vi "BeadTrackerMain.vi"() -> ()   [LabVIEW 2011]
uses:
  qtrk/QTrkLVBinding/QTrkLocalizationType.ctl
  Main/Typedefs/MeasureConfigType.ctl
  Main/Typedefs/MeasureConfigOutputMode.ctl
  qtrk/QTrkLVBinding/QTrkSettings.ctl
  Main/Typedefs/TrackingConfigType.ctl
  qtrk/QTrkLVBinding/QTrkZCommandType.ctl
  Main/ExperimentProgram/ExperimentProgramType.ctl
  Main/ExperimentProgram/ExProgCommandType.ctl
  Main/ExperimentProgram/ExProgCommandEnumType.ctl
  Main/Motors/MotorAxisEnum.ctl
  Main/Motors/MotorPosType.ctl
  Main/Typedefs/XYf.ctl
  Main/Motors/MotorPosFlagsType.ctl
  Main/Camera/GenericCameraConfigType.ctl
  <vilib>/vision/Image Controls.llb/IMAQ Image.ctl
  qtrk/QTrkLVBinding/ResultManagerInstance.ctl
  Main/Typedefs/CmdEnum_UserInterfaceCmd.ctl
  Main/Typedefs/CmdEnum_CameraFrameType.ctl
  Main/GlobalVariables.vi
  Main/Tracking/SemaphoreResultManager.vi
  <vilib>/vision/NI_Vision_Development_Module.lvlib
  <vilib>/Analysis/NI_AALBase.lvlib
panel:
  out "Buffer Image":T1
  in  "Default measure config":T2={"Bead locations"=[{"X"=0, "Y"=0}], "ROI"=80, "Experiment base path"=path "", "Image output subdir"="images", "Output mode"=enum."Track", "Traces output subdir"="traces", "QTrk Settings"={"Image width"=150, "Image height"=150, "Number of threads (CPU based)"=-1, "CUDA Device"=-2, "COM Background correction factor"=0.0, "ZLUT MinRadius"=2.0, "ZLUT Radial sample density"=2.0, "ZLUT Angular sample density"=0.7, "ZLUT ROI Coverage"=1.0, "QI Iterations"=3, "QI MinRadius"=2.0, "QI Radial sample density"=2.0, "QI Angular sample density"=0.7, "QI ROI Coverage"=1.0, "QI Angular Step \nIteration Factor"=1.2, "XCOR Profile Length"=1, "XCOR Profile Width"=128, "XCOR Iterations"=32, "Gaussian 2D Fit Iterations"=2, "Gaussian 2D Sigma (pixels)"=3.0, "Downsample"=0}, "Tracking Config"={"Number of steps"=100, "ZLUT stepsize (um)"=0.05, "Z correction factor"=0.88, "Start piezo Z (um)"=0.0, "Pixel size (nm)"=146.0, "2D Localization Type"=enum."Quadrant Interpolation", "Z Command (None)"=enum."ComputeZ", "Z Piezo scale"=FALSE, "ZLUT Building\nimages per frame"=0}, "Experiment Name"="test", "Program"={"Commands"=[], "Motor Axis accuracy conditions"={"Magnet Z"=0.0, "Magnet rotation"=0.0, "Camera"={"X"=0.0, "Y"=0.0}, "Piezo XY"={"X"=0.0, "Y"=0.0}, "Piezo Z"=0.0, "Coil XY"={"X"=0.0, "Y"=0.0}}, "Axis flags"={"Magnet Z"=FALSE, "Magnet rotation"=FALSE, "Camera"={"X"=FALSE, "Y"=FALSE}, "Piezo XY"={"X"=FALSE, "Y"=FALSE}, "Piezo Z"=FALSE, "Coil XY"={"X"=FALSE, "Y"=FALSE}}}, "ZLUT"=[], "Camera settings"={"Framerate (Hz)"=60, "Exposure time (us)"=5000, "Image size"={"Width"=1280, "Height"=1024}, "Number of buffers"=30}, "Experiment Script"="", "Max frames in memory"=100000, "Save traces as binary"=FALSE, "Pixel Calibration Gain Image"="camera_calib_gain.bin", "Pixel Calibration Offset Image"="camera_calib_offset.bin", "Use pixel calibration images"=FALSE, "Internal camera settings"="", "Trace write interval"=100} {"QTrk Settings"."QI ROI Coverage" format="%_2g"; "QTrk Settings"."QI MinRadius" format="%.2f"; "QTrk Settings"."QI Angular sample density" format="%.3f"; "QTrk Settings"."QI Radial sample density" format="%.2f"; "QTrk Settings"."ZLUT Radial sample density" format="%.2f"; "QTrk Settings"."ZLUT MinRadius" format="%.2f"}
  out "Bead positions":cluster{"X":dbl, "Y":dbl}[](array[cluster])
  in  "Compute fisher accuracy":bool
  out "Offset":sgl[][](array[numeric])
  out "Normalized 1/Gain":sgl[][](array[numeric])
  out "Number of listeners":i32
  out "Running\nexperiment":bool
  out "Cam loop\nupdate speed":dbl
  in  "UpdateTraces":cluster{"ID":dbl}
  in  "UpdateLUT":cluster{"ID":dbl}
  in  "ImageOrResultViewTab":enum32{"Image", "Traces & LUT", "Message Log"}(tab)
  out "Image mean value":sgl(graph)
  in  "Hardware ROI index":i32
  out "Histogram":u32[](graph)
  out "Image":T1(plugin-control)
  out "Frame#":i32
  out "Framerate":dbl format="%#_1f"
  in  "Show image?":bool=TRUE
  in  "Histogram":bool
  out "Minimal Value":sgl
  out "Maximal Value":sgl
  in  "Save image":bool
  out "LUT minimum\nplane index":i32
  in  "Save LUT image":bool
  out "Bead image":u8[][](graph)
  in  "Start frame for trace display":i32(slide) max=9720 scale=0.0..3265.0
  in  "Reference bead#":i32 max=33
  in  "Subtract reference":bool
  in  "Discard bead":bool
  out "Bead XY":sgl[][](graph)
  in  "Bead index":i32 min=0 max=5
  out "Bead Z":sgl[](graph)
  out "Z Lookup Table":sgl[][](graph)
  in  "Number of frames to display":i32=1000 max=33
  out "Bead validity":dbl
  in  "Auto discard":bool
  in  "Minimum bead validity":dbl=1.0
  out "LUT minimum\nplane difference":dbl
  in  "LUT Inspect":bool
  out "Message Log":i32(listbox)
  out "ZLUT":sgl[][][](array[numeric])
  in  "UpdateUI":cluster{"ID":dbl}
  in  "Tab Control":T16(tab)
  out "Camera settings":variant
  in  "Camera settings":bool
  out "Expected location of beadlist:":path
  in  "Load beadlist":bool
  in  "Save beadlist":bool
  in  "ROI":i32=80
  in  "Select beads":bool
  out "Number of beads":i32
  out "LUT location":path
  in  "Load ZLUT":bool
  in  "Save ZLUT":bool
  in  "Save default settings":bool
  in  "Reload default settings":bool
  in  "2D Localization Type":T6
  in  "Pixel size (nm)":sgl=0.88
  in  "Set current piezo Z as start Z":bool
  in  "Edit QTrk settings":bool
  in  "ZLUT Start piezo Z":sgl=0.88
  in  "Number of steps":i32
  in  "Step size (um)":sgl
  in  "Z correction factor":sgl=0.88
  in  "Build ZLUT":bool
  in  "Select QTrk DLL":bool
  out "Settings location:":path
  in  "Use LUT scale for Z":bool=TRUE
  in  "Pixel calibration gain:":path
  in  "Pixel calibration offset:":path
  in  "Use gain/offset \ncorrection?":bool
  out "Mean":dbl format="%0.2f"
  out "Mean":dbl format="%0.2f"
  out "Max":sgl
  out "Min":sgl
  out "Max":sgl
  out "Min":sgl
  out "Gain image size":i32[](array[numeric])
  out "Offset image size":i32[](array[numeric])
  out "St Dev.":dbl format="%0.2f"
  out "St. Dev":dbl format="%0.2f"
  in  "stop":bool
  # "(used for commands with string parameters)"
  # "-2: Use all devices\n-1: Use best device"
  # "If the camera is giving multiple ROIs, this allows you to select the one that is displayed"
  # "Discard bead also discards bead results and bead ZLUT"
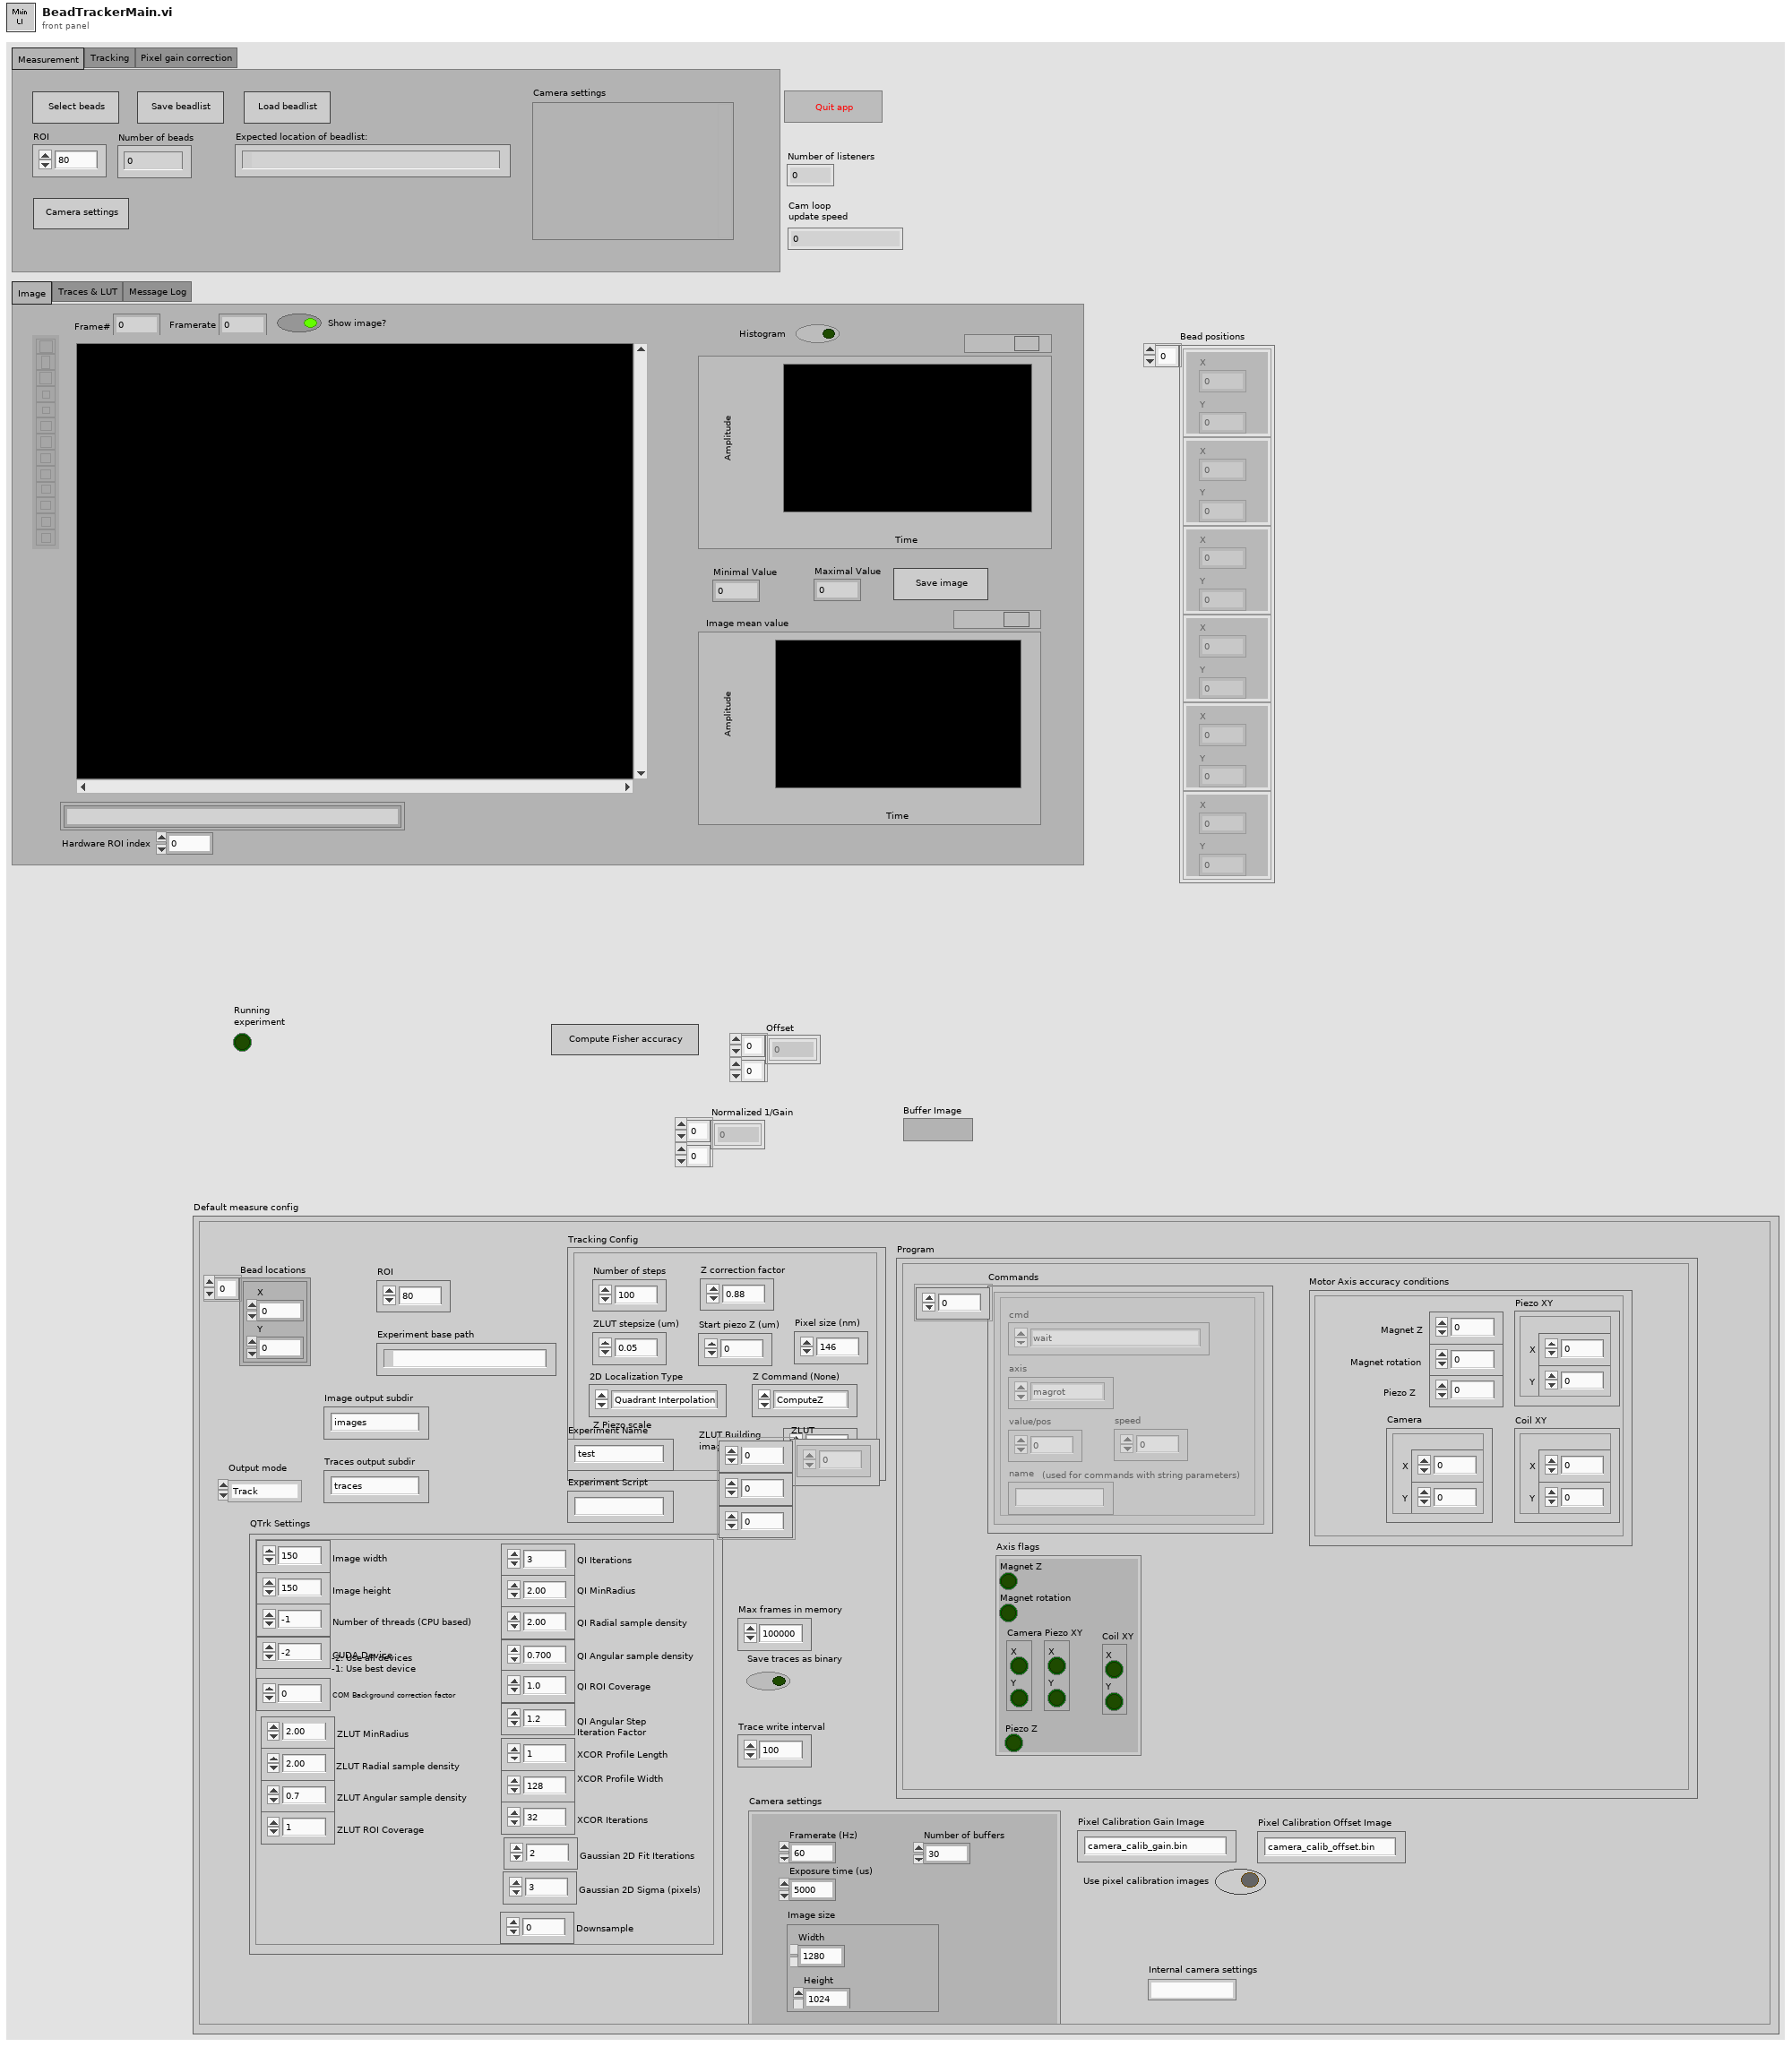
[diagram p1: front panel]
types:
  T1 = typedef "IMAQ Image.ctl" = refnum<image>
  T2 = typedef "MeasureConfigType.ctl" = cluster{"Bead locations":cluster{"X":i32, "Y":i32}[], "ROI":i32, "Experiment base path":path, "Image output subdir":string, "Output mode":T3, "Traces output subdir":string, "QTrk Settings":T4, "Tracking Config":T5, "Experiment Name":string, "Program":T8, "ZLUT":sgl[][][], "Camera settings":T15, "Experiment Script":string, "Max frames in memory":i32, "Save traces as binary":bool, "Pixel Calibration Gain Image":string, "Pixel Calibration Offset Image":string, "Use pixel calibration images":bool, "Internal camera settings":string, "Trace write interval":i32}
  T3 = typedef "MeasureConfigOutputMode.ctl" = enum16{"None", "Track", "SaveImages"}
  T4 = typedef "QTrkSettings.ctl" = cluster{"Image width":i32, "Image height":i32, "Number of threads (CPU based)":i32, "CUDA Device":i32, "COM Background correction factor":sgl, "ZLUT MinRadius":sgl, "ZLUT Radial sample density":sgl, "ZLUT Angular sample density":sgl, "ZLUT ROI Coverage":sgl, "QI Iterations":i32, "QI MinRadius":sgl, "QI Radial sample density":sgl, "QI Angular sample density":sgl, "QI ROI Coverage":sgl, "QI Angular Step \nIteration Factor":sgl, "XCOR Profile Length":i32, "XCOR Profile Width":i32, "XCOR Iterations":i32, "Gaussian 2D Fit Iterations":i32, "Gaussian 2D Sigma (pixels)":sgl, "Downsample":i32}
  T5 = typedef "TrackingConfigType.ctl" = cluster{"Number of steps":i32, "ZLUT stepsize (um)":sgl, "Z correction factor":sgl, "Start piezo Z (um)":sgl, "Pixel size (nm)":sgl, "2D Localization Type":T6, "Z Command (None)":T7, "Z Piezo scale":bool, "ZLUT Building\nimages per frame":i32}
  T6 = typedef "QTrkLocalizationType.ctl" = enum16{"Center-of-Mass", "1D Cross-Correlation", "Quadrant Interpolation", "Gaussian 2D MLE", "QI + ZLUTAlign", "ZLUTAlign", "QI + FourierLUT"}
  T7 = typedef "QTrkZCommandType.ctl" = enum16{"Nothing", "ComputeZ", "BuildRadialZLUT", "BuildImageZLUT", "RadialZLUT+ImageZLUT"}
  T8 = typedef "ExperimentProgramType.ctl" = cluster{"Commands":T9[], "Motor Axis accuracy conditions":T12, "Axis flags":T14}
  T9 = typedef "ExProgCommandType.ctl" = cluster{"cmd":T10, "axis":T11, "value/pos":dbl, "speed":dbl, "name":string}
  T10 = typedef "ExProgCommandEnumType.ctl" = enum16{"wait", "move", "acquire", "idle", "rmove", "when", "section", "stop"}
  T11 = typedef "MotorAxisEnum.ctl" = enum16{"no axis", "magrot", "magpos", "px", "py", "pz", "camx", "camy"}
  T12 = typedef "MotorPosType.ctl" = cluster{"Magnet Z":dbl, "Magnet rotation":dbl, "Camera":T13, "Piezo XY":T13, "Piezo Z":dbl, "Coil XY":T13}
  T13 = typedef "XYf.ctl" = cluster{"X":sgl, "Y":sgl}
  T14 = typedef "MotorPosFlagsType.ctl" = cluster{"Magnet Z":bool, "Magnet rotation":bool, "Camera":cluster{"X":bool, "Y":bool}, "Piezo XY":cluster{"X":bool, "Y":bool}, "Piezo Z":bool, "Coil XY":cluster{"X":bool, "Y":bool}}
  T15 = typedef "GenericCameraConfigType.ctl" = cluster{"Framerate (Hz)":i32, "Exposure time (us)":i32, "Image size":cluster{"Width":i32, "Height":i32}, "Number of buffers":i32}
  T16 = enum32{"Measurement", "Tracking", "Pixel gain correction"}
  T17 = typedef "ResultManagerInstance.ctl" = cluster{"InstancePtr":u64}
  T18 = typedef "CameraInstance.ctl" = cluster{"VI refs":T19, "Camera state":variant}
  T19 = typedef "CameraInterface.ctl" = cluster{"Close":T20, "Get/Set generic config":T21, "Grab":T22, "Show Settings Dialog":T23, "AdjustBeadPos":T24, "Save/load camera settings":T25}
  T20 = typedef "CICloseType.ctl" = refnum<vi>
  T21 = typedef "CIGetSetGenericConfig.ctl" = refnum<vi>
  T22 = typedef "CIGrabType.ctl" = refnum<vi>
  T23 = typedef "CISettingsDlg.ctl" = refnum<vi>
  T24 = typedef "CIAdjustBeadPos.ctl" = refnum<vi>
  T25 = typedef "CISaveLoadSettings.ctl" = refnum<vi>
  T26 = typedef "QueueListType.ctl" = cluster{"Motor In":refnum<queue>, "User Interface Image View":refnum<queue>, "User Interface Camera Control":refnum<queue>, "User Interface Event Notifier":refnum<notifier>, "Initialized?":bool}
  T27 = cluster{"UpdateUI":refnum<user-event>, "UpdateLUT":refnum<user-event>, "UpdateTraces":refnum<user-event>}
  T28 = typedef "CmdEnum_UserInterfaceCmd.ctl" = enum32{"Idle (Use for default)", "ResultTracesUpdated", "MeasureConfigUpdated", "MeasureEnd", "MeasureStart"}
  T29 = typedef "CmdEnum_CameraFrameType.ctl" = enum16{"Full", "HardwareROI", "EndGrabMarker"}
  T30 = typedef "CmdData_NewFrame.ctl" = cluster{"Buffer Image":T1, "Frame #":i32, "Hardware ROI Index":i32, "Timestamp":dbl, "Type":T29}
  T31 = cluster{"histogram":u32[], "Minimal Value":sgl, "Maximal Value":sgl, "Starting Value":sgl, "Interval Width":sgl, "Mean Value":sgl, "Standard  Variation":sgl, "Area (pixels)":i32}
  T32 = enum16{"None", "Normalize", "NormalizeWithoutOffset"}
  T33 = enum16{"big-endian, network order", "native, host order", "little-endian"}
  T34 = enum32{"Invalid", "Standard", "Closed", "Hidden", "Minimized", "Maximized"}
  T35 = typedef "ResultManagerConfig.ctl" = cluster{"Number of beads":i32, "Number of frame info columns":i32, "Result scaling":T36, "Result offset":T36, "Write Interval":i32, "Max frames in memory":i32, "Binary output (1/0)":i8}
  T36 = typedef "XYZf.ctl" = cluster{"X":sgl, "Y":sgl, "Z":sgl}
  T37 = typedef "MotorStateType.ctl" = cluster{"Enabled?":bool, "Current Position":T12, "Update counter":i32}
  T38 = typedef "UserInterfaceEventType.ctl" = cluster{"Type":T28}
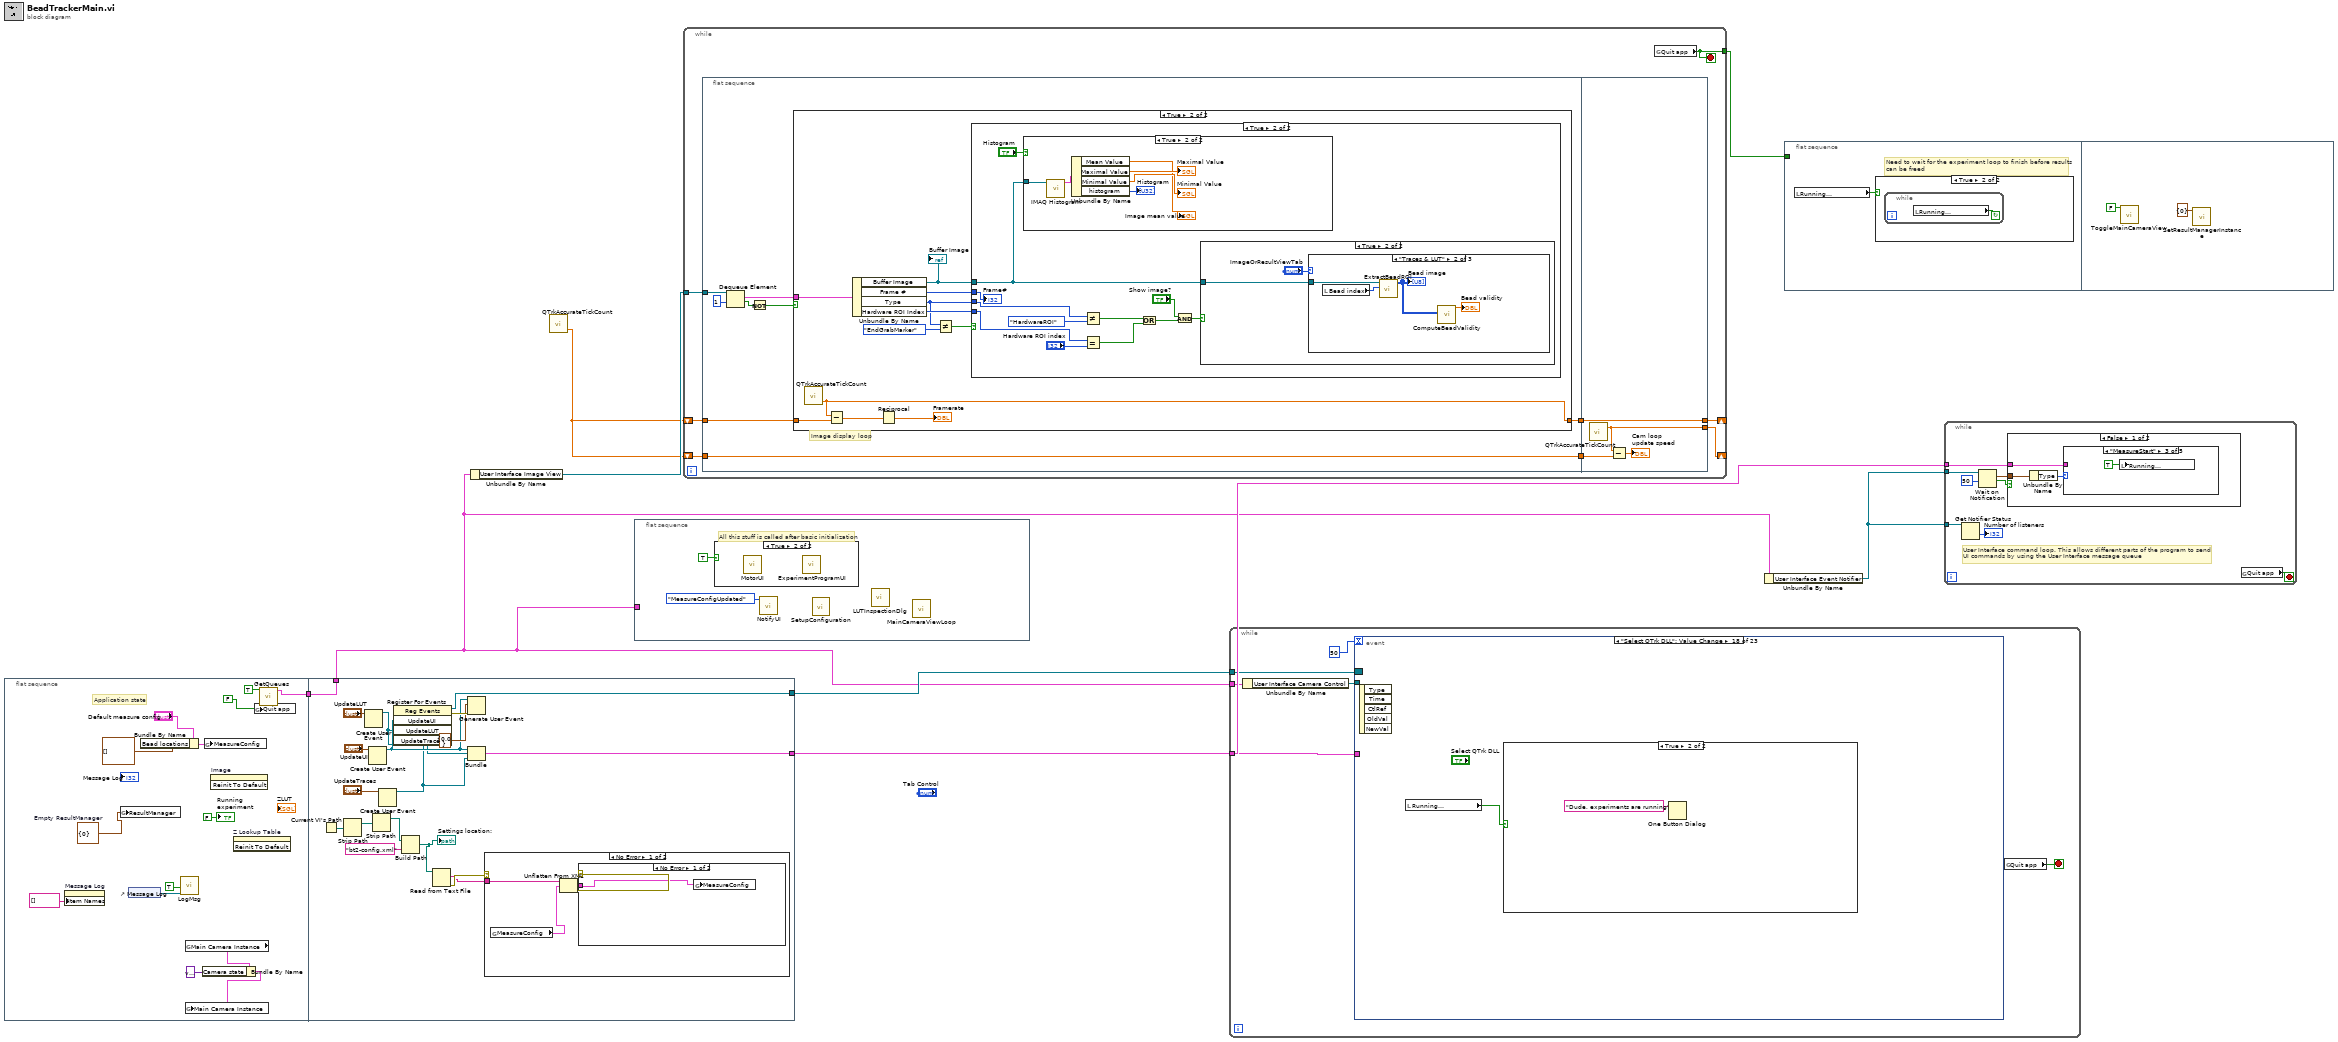
[diagram p0: block diagram]
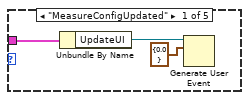
[diagram p3: hidden frame]
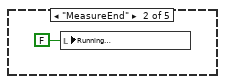
[diagram p4: hidden frame]
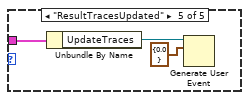
[diagram p6: hidden frame]
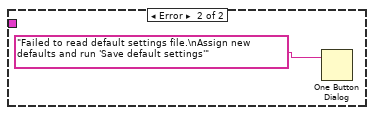
[diagram p9: hidden frame]
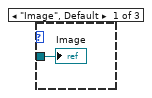
[diagram p15: hidden frame]
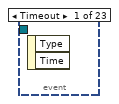
[diagram p17: hidden frame]
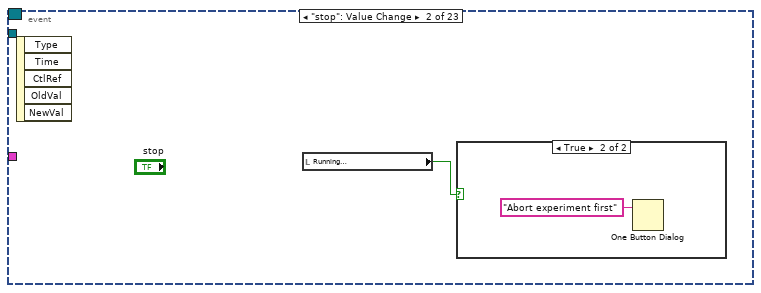
[diagram p18: hidden frame]
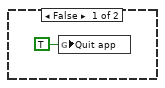
[diagram p19: hidden frame]
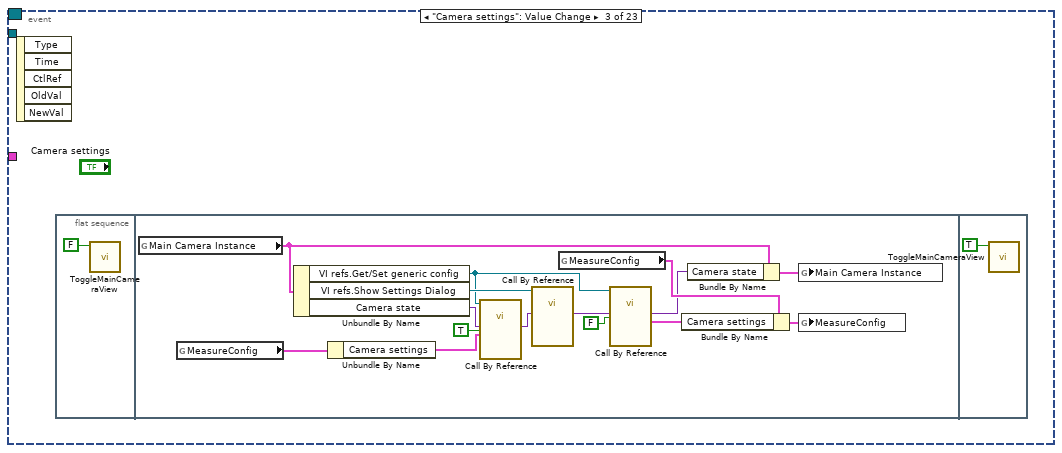
[diagram p20: hidden frame]
diagram:
  n1 = flat-sequence {
    tunnel: [w11] -> w2
    tunnel: [w36] -> w8
    tunnel: [w35] -> w4
    tunnel: w2 -> [w23]
    tunnel: [w23] -> w1
    frame #0 {
      w9 = T17 {"InstancePtr"=0}  # Empty ResultManager
      # "Application state"
      n2 = property on="Message Log" class="LstBox (strict)"("Item Names"=string[] []) -> ()  [unwired: 2 in, 2 out]
      n3 = global write "SemaphoreResultManager.vi" "ResultManager"(w9) -> ()
      n4 = control-ref of="Message Log"() -> (w16:refnum<vi>)
      n5 = Bundle By Name(cluster="Default measure config", "Bead locations"=cluster{"X":i32, "Y":i32}[] []) -> (w19:T2)
      n6 = call "LogMsg.vi"("External listbox\nto add items to"=w16, "Set external listbox"=TRUE) -> ()  [unwired: 10 in]
      n7 = global read "GlobalVariables.vi" "Main Camera Instance"() -> (w14:T18)
      n8 = Bundle By Name(cluster=w14, "Camera state"=variant ("Variant")) -> (w12:T18)
      n9 = global write "GlobalVariables.vi" "Main Camera Instance"(w12) -> ()
      n10 = global write "GlobalVariables.vi" "MeasureConfig"(w19) -> ()
      n11 = invoke on="Image" class="ImageControl" method="Reinit To Default"() -> ()  [unwired: 3 in, 3 out]
      n12 = invoke on="Z Lookup Table" class="IntGraph (strict)" method="Reinit To Default"() -> ()  [unwired: 3 in, 3 out]
      n13 = global write "GlobalVariables.vi" "Quit app"(FALSE ("Quit app")) -> ()
      n14 = call "GetQueues.vi"("create new? (F)"=TRUE ("create new?")) -> ("Queue List"=w11:T26)  [unwired: 9 in, 1 out]
      "Running\nexperiment" <- FALSE ("Running\nexperiment")
    }
    frame #1 {
      n15 = Current VI's Path() -> (path=w29:path)
      n16 = Strip Path(path=w29) -> (stripped path=w28:path)  [unwired: 1 out]
      n17 = Create User Event(user event datatype="UpdateLUT") -> (user event=w33:refnum<user-event>)  [unwired: 1 in, 1 out]
      n18 = Create User Event(user event datatype="UpdateUI") -> (user event=w38:refnum<user-event>)  [unwired: 1 in, 1 out]
      n19 = Strip Path(path=w28) -> (stripped path=w27:path)  [unwired: 1 out]
      n20 = Create User Event(user event datatype="UpdateTraces") -> (user event=w31:refnum<user-event>)  [unwired: 1 in, 1 out]
      n21 = register-events(w38, w33, w31) -> (reference out=w36:refnum<event-registration>, error out=w40:errorcluster)  [unwired: 2 in]
      n22 = Build Path(base path=w27, name or relative path="bt2-config.xml") -> (appended path=w26:path)
      "Settings location:" <- w26
      n23 = Read from Text File(file (use dialog)=w26) -> (text=w24:string, error out=w25:errorcluster)  [unwired: 3 in, 2 out]
      n24 = Generate User Event(user event=w38, event data cluster=cluster{"ID":dbl} {"ID"=0.0} ("event data"), error in=w40) -> ()  [unwired: 2 out]
      n25 = Bundle("UpdateUI"=w38, "UpdateLUT"=w33, "UpdateTraces"=w31) -> (w35:T27)  [unwired: 1 in]
      n26 = case shown="No Error" w25 {
        tunnel: w24 -> [w42 _]
        frame No Error {
          n27 = global read "GlobalVariables.vi" "MeasureConfig"() -> (w41:T2)
          n28 = Unflatten From XML(xml string=w42, type=w41) -> (value=w43:T2, error out=w44:errorcluster)  [unwired: 1 in]
          n29 = case shown="No Error" w44 {
            tunnel: w43 -> [w45 _]
            frame No Error {
              n30 = global write "GlobalVariables.vi" "MeasureConfig"(w45) -> ()
            }
            frame Error {
              n31 = One Button Dialog(message="Failed to read default settings file.\nAssign new defaults and run 'Save default settings'" ("msg")) -> ()  [unwired: 1 in, 1 out]
            }
          }
        }
        frame Error {
        }
      }
    }
  }
  n32 = Unbundle By Name(w1) -> ("User Interface Image View"=w7:refnum<queue>)
  n33 = call "QTrkAccurateTickCount.vi"() -> ("seconds"=w6:dbl)  [unwired: 2 in, 1 out]
  n34 = flat-sequence {
    tunnel: w1 -> [_]
    frame #0 {
      # "All this stuff is called after basic initialization"
      n35 = case shown="True" TRUE {
        frame False {
        }
        frame True {
          n36 = call "MotorUI.vi"() -> ()  [unwired: 12 in]
          n37 = call "ExperimentProgramUI.vi"() -> ()  [unwired: 12 in]
        }
      }
      n38 = call "NotifyUI.vi"("User Interface Commands"=CmdEnum_UserInterfaceCmd."MeasureConfigUpdated") -> ()  [unwired: 11 in]
      n39 = call "SetupConfiguration.vi"() -> ()  [unwired: 12 in]
      n40 = call "LUTInspectionDlg.vi"() -> ()  [unwired: 12 in]
      n41 = call "MainCameraViewLoop.vi"() -> ()  [unwired: 12 in]
    }
  }
  n42 = while {
    tunnel: w7 -> [w56]
    shift-right: [w54] -> _
    shift-left: w6 -> [w55]
    shift-right: [w50] -> _
    shift-left: w6 -> [w51]
    tunnel: [w49] -> w5
    stop <- w49 stop-if-true
    n43 = flat-sequence {
      tunnel: [w64] -> w53
      tunnel: w56 -> [w59]
      tunnel: [w57] -> w52
      tunnel: w51 -> [w64]
      tunnel: w55 -> [w58]
      tunnel: w53 -> [w105]
      tunnel: [w103] -> w54
      tunnel: w52 -> [w103]
      tunnel: [w102] -> w50
      frame #0 {
        # "Image display loop"
        n44 = Dequeue Element(queue=w59, timeout in ms (-1)=1) -> (element=w60:T30, timed out?=w62:bool)  [unwired: 1 in, 2 out]
        n45 = Not(x=w62) -> (.not. x?=w61:bool)
        n46 = case shown="True" w61 {
          tunnel: w60 -> [_ w72]
          tunnel: w58 -> [w65 w76]
          tunnel: [w65 w75] -> w57
          frame False {
          }
          frame True {
            n47 = call "QTrkAccurateTickCount.vi"() -> ("seconds"=w75:dbl)  [unwired: 2 in, 1 out]
            n48 = Subtract(x=w75, y=w76) -> (x-y=w74:dbl)
            n49 = Unbundle By Name(w72) -> ("Buffer Image"=w71:T1, "Frame #"=w66:i32, "Type"=w69:T29, "Hardware ROI Index"=w70:i32)
            "Buffer Image" <- w71
            n50 = Reciprocal(x=w74) -> (1/x=→"Framerate":dbl)
            n51 = Not Equal?(x=w69, y=CmdEnum_CameraFrameType."EndGrabMarker") -> (x != y?=w67:bool)
            n52 = case shown="True" w67 {
              tunnel: w71 -> [_ w87]
              tunnel: w70 -> [_ w85]
              tunnel: w69 -> [_ w79]
              tunnel: w66 -> [_ w80]
              frame False {
              }
              frame True {
                n53 = case shown="True" "Histogram" {
                  tunnel: w87 -> [_ w94]
                  frame False {
                  }
                  frame True {
                    n54 = call "IMAQ Histogram"("Image"=w94) -> ("Histogram Report"=w93:T31)  [unwired: 9 in, 1 out]
                    n55 = Unbundle By Name(w93) -> ("Mean Value"=→"Image mean value":sgl, "Maximal Value"=→"Maximal Value":sgl, "Minimal Value"=→"Minimal Value":sgl, "histogram"=→"Histogram":u32[])
                  }
                }
                n56 = Not Equal?(x=w79, y=CmdEnum_CameraFrameType."HardwareROI") -> (x != y?=w77:bool)
                n57 = Equal?(x=w85, y="Hardware ROI index") -> (x = y?=w83:bool)
                n58 = Or(x=w77, y=w83) -> (x .or. y?=w82:bool)
                n59 = And(x="Show image?", y=w82) -> (x .and. y?=w81:bool)
                n60 = case shown="True" w81 {
                  tunnel: w87 -> [_ w95]
                  frame False {
                  }
                  frame True {
                    n61 = case shown="\"Traces & LUT\"" "ImageOrResultViewTab" {
                      tunnel: w95 -> [w97 w101 _]
                      frame "Image", Default {
                        "Image" <- w97
                      }
                      frame "Traces & LUT" {
                        n62 = local read "Bead index"() -> (w100:i32)
                        n63 = call "ExtractBeadROI.vi"("Bead index"=w100, "Image"=w101) -> ("Image Pixels (U8)"=w99:u8[][])  [unwired: 9 in]
                        "Bead image" <- w99
                        n64 = call "ComputeBeadValidity.vi"("Image Pixels (U8)"=w99) -> ("Bead validity"=→"Bead validity":dbl)  [unwired: 10 in]
                      }
                      frame "Message Log" {
                      }
                    }
                  }
                }
                "Frame#" <- w80
              }
            }
          }
        }
      }
      frame #1 {
        n65 = call "QTrkAccurateTickCount.vi"() -> ("tick count (ms)"=w102:dbl)  [unwired: 2 in, 1 out]
        n66 = Subtract(x=w102, y=w105) -> (x-y=→"Cam loop\nupdate speed":dbl)
      }
    }
    n67 = global read "GlobalVariables.vi" "Quit app"() -> (w49:bool)
  }
  n68 = while {
    tunnel: w1 -> [w110]
    tunnel: w8 -> [w108]
    tunnel: w4 -> [w107]
    stop <- w106 stop-if-true
    n69 = Unbundle By Name(w110) -> ("User Interface Camera Control"=w109:refnum<queue>)
    n70 = event shown="[17] \"Select QTrk DLL\": Value Change" {
      selector: w108 -> [_ _ _ _ _ _ _ _ _ _ _ _ _ _ _ _ _ _ _ _ _ _ _]
      dyn-events: _ -> [_ _ _ _ _ _ _ _ _ _ _ _ _ _ _ _ _ _ _ _ _ _ _]
      timeout: 50 -> [_ _ _ _ _ _ _ _ _ _ _ _ _ _ _ _ _ _ _ _ _ _ _]
      tunnel: w109 -> [_ _ _ _ _ _ _ _ _ _ _ _ _ _ _ _ _ _ _ _ _ _ _]
      tunnel: w107 -> [_ _ _ w132 _ _ _ w219 _ _ _ _ w249 w263 _ _ w277 _ w321 _ _ _ w347]
      event Timeout {
        n71 = event-data() -> ()  [unwired: 1 in, 2 out]
      }
      event "stop": Value Change {
        n72 = event-data() -> ()  [unwired: 1 in, 5 out]
        n73 = local read "Running\nexperiment"() -> (w112:bool)
        n74 = case shown="True" w112 {
          frame False {
            n75 = global write "GlobalVariables.vi" "Quit app"(TRUE ("Quit app")) -> ()
          }
          frame True {
            n76 = One Button Dialog(message="Abort experiment first") -> ()  [unwired: 1 in, 1 out]
          }
        }
      }
      event "Camera settings": Value Change {
        n77 = event-data() -> ()  [unwired: 1 in, 5 out]
        n78 = flat-sequence {
          frame #0 {
            n79 = call "ToggleMainCameraView.vi"("Enable? (T)"=FALSE) -> ()  [unwired: 11 in]
          }
          frame #1 {
            n80 = global read "GlobalVariables.vi" "Main Camera Instance"() -> (w129:T18)
            n81 = global read "GlobalVariables.vi" "MeasureConfig"() -> (w119:T2)
            n82 = Unbundle By Name(w129) -> ("VI refs.Get/Set generic config"=w121:T21, "VI refs.Show Settings Dialog"=w130:T23, "Camera state"=w120:variant)
            n83 = Unbundle By Name(w119) -> ("Camera settings"=w118:T15)
            n84 = call-by-ref "?"(reference=w121, "Set? (F)"=TRUE, "GenericCameraConfig"=w118, "Camera state"=w120) -> ("Camera state (out)"=w117:variant)  [unwired: 8 in, 3 out]
            n85 = call-by-ref "?"(reference=w130, "Camera state"=w117) -> ("Camera state (out)"=w127:variant)  [unwired: 11 in, 2 out]
            n86 = global read "GlobalVariables.vi" "MeasureConfig"() -> (w125:T2)
            n87 = call-by-ref "?"(reference=w121, "Set? (F)"=FALSE, "Camera state"=w127) -> ("GenericCameraConfig (out)"=w124:T15, "Camera state (out)"=w123:variant)  [unwired: 9 in, 2 out]
            n88 = Bundle By Name(cluster=w125, "Camera settings"=w124) -> (w122:T2)
            n89 = Bundle By Name(cluster=w129, "Camera state"=w123) -> (w128:T18)
            n90 = global write "GlobalVariables.vi" "Main Camera Instance"(w128) -> ()
            n91 = global write "GlobalVariables.vi" "MeasureConfig"(w122) -> ()
          }
          frame #2 {
            n92 = call "ToggleMainCameraView.vi"("Enable? (T)"=TRUE) -> ()  [unwired: 11 in]
          }
        }
      }
      event "Select beads": Value Change {
        n93 = event-data() -> ()  [unwired: 1 in, 5 out]
        n94 = flat-sequence {
          tunnel: w132 -> [w134]
          frame #0 {
            n95 = local read "Image"() -> (w133:T1)
            n96 = call "SelectBeads.vi"("Input image"=w133) -> ()  [unwired: 11 in]
          }
          frame #1 {
            n97 = Unbundle By Name(w134) -> ("UpdateUI"=w135:refnum<user-event>)
            n98 = Generate User Event(user event=w135, event data cluster=cluster{"ID":dbl} {"ID"=0.0} ("event data")) -> ()  [unwired: 1 in, 2 out]
          }
        }
      }
      event "ROI", "Number of steps", "Step size (um)", "Z correction factor", "ZLUT Start piezo Z", "Pixel size (nm)", "Use gain/offset \ncorrection?", "Pixel calibration gain:", "Pixel calibration offset:", "Use LUT scale for Z": Value Change {
        n99 = event-data() -> ()  [unwired: 1 in, 5 out]
        n100 = global read "GlobalVariables.vi" "MeasureConfig"() -> (w146:T2)
        n101 = Path To String(path="Pixel calibration gain:") -> (string=w138:string)
        n102 = Path To String(path="Pixel calibration offset:") -> (string=w139:string)
        n103 = Bundle By Name(cluster=w146, "ROI"="ROI", "Tracking Config.Number of steps"="Number of steps", "Tracking Config.ZLUT stepsize (um)"="Step size (um)", "Tracking Config.Z correction factor"="Z correction factor", "Tracking Config.Start piezo Z (um)"="ZLUT Start piezo Z", "Tracking Config.Pixel size (nm)"="Pixel size (nm)", "Tracking Config.2D Localization Type"="2D Localization Type", "Pixel Calibration Gain Image"=w138, "Pixel Calibration Offset Image"=w139, "Use pixel calibration images"="Use gain/offset \ncorrection?", "Tracking Config.Z Piezo scale"="Use LUT scale for Z") -> (w147:T2)
        n104 = global write "GlobalVariables.vi" "MeasureConfig"(w147) -> ()
        n105 = call "NotifyUI.vi"("User Interface Commands"=CmdEnum_UserInterfaceCmd."MeasureConfigUpdated") -> ()  [unwired: 11 in]
      }
      event "Save default settings", "Reload default settings": Value Change {
        n106 = event-data() -> ()  [unwired: 1 in, 5 out]
        n107 = local read "Settings location:"() -> (w153:path)
        n108 = case shown="True" "Reload default settings" {
          tunnel: w153 -> [w165 w171]
          frame False {
            n109 = global read "GlobalVariables.vi" "Main Camera Instance"() -> (w162:T18)
            n110 = global read "GlobalVariables.vi" "MeasureConfig"() -> (w158:T2)
            n111 = Unbundle By Name(w162) -> ("VI refs.Save/load camera settings"=w161:T25, "Camera state"=w160:variant)
            n112 = call-by-ref "?"(reference=w161, "Save?"=FALSE, "Camera data"=w160) -> ("Serialized data (out)"=w156:string)  [unwired: 9 in, 3 out]
            n113 = Bundle By Name(cluster=w158, "Internal camera settings"=w156) -> (w157:T2)
            n114 = Bundle By Name(cluster=w157, "ZLUT"=sgl[][][] []) -> (w155:T2)
            n115 = Flatten To XML(anything=w155) -> (xml string=w164:string)
            n116 = Write to Text File(file (use dialog)=w165, text=w164) -> ()  [unwired: 2 in, 3 out]
          }
          frame True {
            n117 = global read "GlobalVariables.vi" "MeasureConfig"() -> (w166:T2)
            n118 = global read "GlobalVariables.vi" "Main Camera Instance"() -> (w168:T18)
            n119 = Read from Text File(file (use dialog)=w171) -> (text=w170:string)  [unwired: 3 in, 3 out]
            n120 = Unflatten From XML(xml string=w170, type=w166) -> (value=w167:T2, error out=w169:errorcluster)  [unwired: 1 in]
            n121 = case shown="No Error" w169 {
              tunnel: w168 -> [w173 _]
              tunnel: w167 -> [w172 _]
              frame No Error {
                n122 = flat-sequence {
                  tunnel: w172 -> [w178]
                  frame #0 {
                    n123 = global write "GlobalVariables.vi" "MeasureConfig"(w178) -> ()
                  }
                  frame #1 {
                    n124 = call "NotifyUI.vi"("User Interface Commands"=CmdEnum_UserInterfaceCmd."MeasureConfigUpdated") -> ()  [unwired: 11 in]
                  }
                }
                n125 = Unbundle By Name(w173) -> ("VI refs.Save/load camera settings"=w175:T25, "Camera state"=w174:variant)
                n126 = Unbundle By Name(w172) -> ("Internal camera settings"=w177:string)
                n127 = call-by-ref "?"(reference=w175, "Save?"=TRUE, "Serialized data"=w177, "Camera data"=w174) -> ()  [unwired: 8 in, 4 out]
              }
              frame Error {
              }
            }
          }
        }
      }
      event User Event; "Reference bead#", "Subtract reference", "Start frame for trace display", "Number of frames to display": Value Change {
        w193 = 0 ("lower limit")
        n128 = event-data() -> ()  [unwired: 1 in, 2 out]
        n129 = call "LockUnlockResultManager.vi"() -> ("ResultManager"=w180:T17)  [unwired: 9 in, 2 out]
        n130 = call "RMGetConfig.vi"("ResultManager"=w180) -> ("config"=w186:T35)  [unwired: 9 in, 1 out]
        n131 = Unbundle By Name(w186) -> ("Number of beads"=w185:i32)
        n132 = Unbundle By Name(w180) -> ("InstancePtr"=w194:u64)
        n133 = Decrement(x=w185) -> (x-1=w192:i32)
        n134 = In Range and Coerce(upper limit=w192, x="Bead index", lower limit=w193) -> (In Range?=w190:bool)  [unwired: 1 out]
        n135 = In Range and Coerce(upper limit=w192, x="Reference bead#", lower limit=w193) -> (In Range?=w184:bool)  [unwired: 1 out]
        n136 = Not Equal To 0?(x=w194) -> (x != 0?=w191:bool)
        n137 = Not(x="Subtract reference") -> (.not. x?=w182:bool)
        n138 = Or(x=w184, y=w182) -> (x .or. y?=w181:bool)
        n139 = Compound Arithmetic op=AND(w191, w190, w181) -> (w189:bool)
        n140 = case shown="False" w189 {
          tunnel: w180 -> [_ w203]
          tunnel: "Reference bead#" -> [_ w199]
          tunnel: "Bead index" -> [_ w198]
          tunnel: "Subtract reference" -> [_ w197]
          frame False {
            n141 = call "LockUnlockResultManager.vi"("Lock? (T)"=FALSE) -> ()  [unwired: 8 in, 3 out]
          }
          frame True {
            n142 = flat-sequence {
              tunnel: w203 -> [w214]
              tunnel: [w213] -> w202
              tunnel: [w211] -> w201
              tunnel: w199 -> [w210]
              tunnel: w198 -> [w209]
              tunnel: w197 -> [w205]
              tunnel: [FALSE ("Lock? (T)")] -> w196
              frame #0 {
                n143 = call "RMGetFrameCounters.vi"("ResultManager"=w214) -> ("ResultManager (out)"=w212:T17, "endFrame"=w208:i32)  [unwired: 7 in, 6 out]
                n144 = Subtract(x=w208, y="Number of frames to display") -> (x-y=w206:i32)
                n145 = call "GenerateTracePlotData.vi"("Reference bead#"=w210, "ResultManager"=w212, "Subtract reference"=w205, "Number of frames to display"="Number of frames to display", "Start frame for trace display"=w206, "Bead index"=w209) -> ("Bead Z"=w213:sgl[], "Bead XY"=w211:sgl[][])  [unwired: 4 in]
              }
            }
            n146 = Transpose 2D Array(2D array=w201) -> (transposed array=→"Bead XY":sgl[][])
            n147 = call "LockUnlockResultManager.vi"("Lock? (T)"=w196) -> ()  [unwired: 8 in, 3 out]
            "Bead Z" <- w202
          }
        }
      }
      event "Bead index": Value Change {
        n148 = event-data() -> ()  [unwired: 1 in, 5 out]
        n149 = Unbundle By Name(w219) -> ("UpdateLUT"=w218:refnum<user-event>, "UpdateTraces"=w217:refnum<user-event>)
        n150 = Generate User Event(user event=w218, event data cluster=cluster{"ID":dbl} {"ID"=0.0} ("event data")) -> ()  [unwired: 1 in, 2 out]
        n151 = Generate User Event(user event=w217, event data cluster=cluster{"ID":dbl} {"ID"=0.0} ("event data")) -> ()  [unwired: 1 in, 2 out]
      }
      event "Discard bead": Value Change {
        n152 = event-data() -> ()  [unwired: 1 in, 5 out]
        n153 = local read "Running\nexperiment"() -> (w220:bool)
        n154 = case shown="False" w220 {
          frame False {
            n155 = flat-sequence {
              frame #0 {
                n156 = local read "Bead index"() -> (w221:i32)
                n157 = call "DiscardBead.vi"("Bead index"=w221) -> ()  [unwired: 11 in]
              }
              frame #1 {
                n158 = global read "GlobalVariables.vi" "MeasureConfig"() -> (w227:T2)
                n159 = Unbundle By Name(w227) -> ("Bead locations"=w226:cluster{"X":i32, "Y":i32}[])
                n160 = Array Size(array=w226) -> (size(s)=w224:i32)
                n161 = local read "Bead index"() -> (w225:i32)
                n162 = Decrement(x=w224) -> (x-1=w223:i32)
                n163 = Max & Min(x=w225, y=w223) -> (min(x,y)=w222:i32)  [unwired: 1 out]
                n164 = local write "Bead index"(w222) -> ()
              }
            }
          }
          frame True {
            n165 = One Button Dialog(message="Can't discard bead while doing experiment") -> ()  [unwired: 1 in, 1 out]
          }
        }
      }
      event "Compute fisher accuracy": Value Change {
        n166 = event-data() -> ()  [unwired: 1 in, 5 out]
        n167 = global read "GlobalVariables.vi" "MeasureConfig"() -> (w229:T2)
        n168 = Unbundle By Name(w229) -> ("ZLUT"=w230:sgl[][][])
        n169 = Empty Array?(array=w230) -> (empty?=w231:bool)
        n170 = case shown="False" w231 {
          tunnel: w229 -> [w234 _]
          frame False {
            n171 = local read "Bead index"() -> (w232:i32)
            n172 = call "ComputeFisherMatrixFromLUT.vi"("Show as dialog?"=TRUE, "MeasureConfig"=w234, "Bead index"=w232) -> ()  [unwired: 8 in, 1 out]
          }
          frame True {
          }
        }
      }
      event "Save image": Value Change {
        n173 = event-data() -> ()  [unwired: 1 in, 5 out]
        n174 = local read "Image"() -> (w239:T1)
        n175 = call "File Dialog"("prompt"="Select output filename:") -> ("selected path"=w235:path, "cancelled"=w237:bool)  [unwired: 11 in, 2 out]
        n176 = call "IMAQ ImageToArray"("Image"=w239) -> ("Image Pixels (U8)"=w236:u8[][])  [unwired: 3 in, 4 out]
        n177 = case shown="False" w237 {
          tunnel: w236 -> [w240 _]
          tunnel: w235 -> [w241 _]
          frame False {
            n178 = call "WriteArrayAsImage.vi"("Data"=w240, "File Path"=w241) -> ()  [unwired: 10 in]
          }
          frame True {
          }
        }
      }
      event "Save LUT image": Value Change {
        n179 = event-data() -> ()  [unwired: 1 in, 5 out]
        n180 = local read "Z Lookup Table"() -> (w242:sgl[][])
        n181 = call "File Dialog2"("prompt"="Select output filename:") -> ("selected path"=w243:path, "cancelled"=w244:bool)  [unwired: 11 in, 2 out]
        n182 = case shown="False" w244 {
          tunnel: w243 -> [w248 _]
          tunnel: w242 -> [w247 _]
          frame False {
            n183 = call "WriteArrayAsImage.vi"("Data"=w247, "File Path"=w248, "Normalize Mode"=T32."Normalize") -> ()  [unwired: 9 in]
          }
          frame True {
          }
        }
      }
      event "Build ZLUT": Value Change {
        n184 = event-data() -> ()  [unwired: 1 in, 5 out]
        n185 = flat-sequence {
          tunnel: [w254] -> w250
          tunnel: w250 -> [w260]
          tunnel: w249 -> [w256]
          frame #0 {
            n186 = call "QTrkCheckForDLL.vi"() -> ()  [unwired: 12 in]
            n187 = call "ToggleMainCameraView.vi"("Enable? (T)"=FALSE) -> ()  [unwired: 11 in]
          }
          frame #1 {
            n188 = global read "GlobalVariables.vi" "MeasureConfig"() -> (w253:T2)
            n189 = call "BuildZLUT.vi"("MeasureConfig"=w253) -> ("ZLUT"=w254:sgl[][][])  [unwired: 9 in, 1 out]
            n190 = Bundle By Name(cluster=w253, "ZLUT"=w254) -> (w252:T2)
            n191 = local write "ZLUT"(w254) -> ()
            n192 = global write "GlobalVariables.vi" "MeasureConfig"(w252) -> ()
          }
          frame #2 {
            n193 = Array Size(array=w260) -> (size(s)=w259:i32[])
            n194 = Index Array(array=w259, index=0) -> ()  [unwired: 1 out]
            n195 = call "ToggleMainCameraView.vi"() -> ()  [unwired: 12 in]
            n196 = Unbundle By Name(w256) -> ("UpdateLUT"=w255:refnum<user-event>)
            n197 = Generate User Event(user event=w255, event data cluster=cluster{"ID":dbl} {"ID"=0.0} ("event data")) -> ()  [unwired: 1 in, 2 out]
          }
        }
      }
      event "Set current piezo Z as start Z": Value Change {
        n198 = event-data() -> ()  [unwired: 1 in, 5 out]
        n199 = global read "GlobalVariables.vi" "MotorState"() -> (w267:T37)
        n200 = Unbundle By Name(w267) -> ("Current Position.Piezo Z"=w266:dbl)
        n201 = global read "GlobalVariables.vi" "MeasureConfig"() -> (w262:T2)
        n202 = Unbundle By Name(w263) -> ("UpdateUI"=w265:refnum<user-event>)
        n203 = Generate User Event(user event=w265, event data cluster=cluster{"ID":dbl} {"ID"=0.0} ("event data")) -> ()  [unwired: 1 in, 2 out]
        n204 = Bundle By Name(cluster=w262, "Tracking Config.Start piezo Z (um)"=w266) -> (w261:T2)
        n205 = global write "GlobalVariables.vi" "MeasureConfig"(w261) -> ()
      }
      event "Edit QTrk settings": Value Change {
        n206 = event-data() -> ()  [unwired: 1 in, 5 out]
        n207 = global read "GlobalVariables.vi" "MeasureConfig"() -> (w270:T2)
        n208 = Unbundle By Name(w270) -> ("QTrk Settings"=w272:T4, "ROI"=w268:i32)
        n209 = call "EditQTrkSettingsDialog.vi"("ROI"=w268, "Settings"=w272) -> ("Settings (output)"=w271:T4)  [unwired: 9 in]
        n210 = Bundle By Name(cluster=w270, "QTrk Settings"=w271) -> (w269:T2)
        n211 = global write "GlobalVariables.vi" "MeasureConfig"(w269) -> ()
      }
      event "Save ZLUT": Value Change {
        n212 = event-data() -> ()  [unwired: 1 in, 5 out]
        n213 = global read "GlobalVariables.vi" "MeasureConfig"() -> (w276:T2)
        n214 = Unbundle By Name(w276) -> ("ZLUT"=w274:sgl[][][])
        n215 = call "GetExperimentPaths.vi"("MeasureConfig"=w276) -> ("[base]\\[expname].radialzlut"=w275:path)  [unwired: 6 in, 8 out]
        n216 = Write to Binary File(file (use dialog)=w275, data=w274, 9:T33."little-endian" ("byte order (0:big-endian, network order)")) -> ()  [unwired: 3 in, 3 out]
      }
      event "Load ZLUT": Value Change {
        n217 = event-data() -> ()  [unwired: 1 in, 5 out]
        n218 = global read "GlobalVariables.vi" "MeasureConfig"() -> (w283:T2)
        n219 = call "GetExperimentPaths.vi"("MeasureConfig"=w283) -> ("[base]\\[expname].radialzlut"=w282:path)  [unwired: 6 in, 8 out]
        n220 = Read from Binary File(5:sgl[][][] [] ("ZLUT"), 9:T33."little-endian" ("byte order (0:big-endian, network order)"), 11:w282) -> (2:w278:sgl[][][])  [unwired: 3 in, 3 out]
        n221 = call "CheckZLUTDimensions.vi"("ZLUT"=w278, "MeasureConfig"=w283) -> ("OK?"=w279:bool)  [unwired: 9 in]
        n222 = case shown="True" w279 {
          tunnel: w278 -> [_ w288]
          tunnel: w277 -> [_ w284]
          frame False {
          }
          frame True {
            n223 = Unbundle By Name(w284) -> ("UpdateLUT"=w286:refnum<user-event>)
            n224 = global read "GlobalVariables.vi" "MeasureConfig"() -> (w289:T2)
            n225 = Generate User Event(user event=w286, event data cluster=cluster{"ID":dbl} {"ID"=0.0} ("event data")) -> ()  [unwired: 1 in, 2 out]
            n226 = Bundle By Name(cluster=w289, "ZLUT"=w288) -> (w287:T2)
            n227 = global write "GlobalVariables.vi" "MeasureConfig"(w287) -> ()
          }
        }
      }
      event "Select QTrk DLL": Value Change {
        n228 = event-data() -> ()  [unwired: 1 in, 5 out]
        n229 = local read "Running\nexperiment"() -> (w290:bool)
        n230 = case shown="True" w290 {
          frame False {
            n231 = flat-sequence {
              frame #0 {
                # "The ResultManager can still point to memory in the old DLL"
                n232 = call "SetResultManagerInstance.vi"("ResultManager"=T17 {"InstancePtr"=0}) -> ()  [unwired: 11 in]
              }
              frame #1 {
                n233 = call "QTrkSelectDLLDialog.vi"() -> ()  [unwired: 11 in, 1 out]
              }
            }
          }
          frame True {
            n234 = One Button Dialog(message="Dude, experiments are running") -> ()  [unwired: 1 in, 1 out]
          }
        }
      }
      event User Event {
        n235 = event-data() -> ()  [unwired: 1 in, 4 out]
        n236 = Unbundle By Name(w321) -> ("UpdateLUT"=w320:refnum<user-event>)
        n237 = global read "GlobalVariables.vi" "MeasureConfig"() -> (w315:T2)
        n238 = Generate User Event(user event=w320, event data cluster=cluster{"ID":dbl} {"ID"=0.0} ("event data")) -> ()  [unwired: 1 in, 2 out]
        n239 = Unbundle By Name(w315) -> ("Bead locations"=w294:cluster{"X":i32, "Y":i32}[], "ROI"=w331:i32, "Tracking Config"=w330:T5, "Tracking Config.2D Localization Type"=w322:T6, "Camera settings"=→"Camera settings":T15)  [unwired: 2 out]
        "Bead positions" <- w294
        n240 = call "GetExperimentPaths.vi"("MeasureConfig"=w315) -> ("[base]\\beadlist.txt"=→"Expected location of beadlist:":path, "[base]\\[expname].radialzlut"=→"LUT location":path)  [unwired: 6 in, 7 out]
        n241 = property on="ROI" class="DigNum (strict)"("Value"=w331) -> ()  [unwired: 2 in, 2 out]
        n242 = Unbundle By Name(w330) -> ("Number of steps"=w329:i32, "ZLUT stepsize (um)"=w328:sgl, "Z correction factor"=w327:sgl, "Start piezo Z (um)"=w325:sgl, "Pixel size (nm)"=w323:sgl, "Z Piezo scale"=w293:bool)
        n243 = local write "2D Localization Type"(w322) -> ()
        n244 = Array Size(array=w294) -> (size(s)=w318:i32)
        "Number of beads" <- w318
        n245 = Unbundle By Name(w315) -> ("Pixel Calibration Gain Image"=w312:string, "Pixel Calibration Offset Image"=w313:string, "Use pixel calibration images"=w314:bool)
        n246 = Decrement(x=w318) -> (x-1=w316:i32)
        n247 = property on="Number of steps" class="DigNum (strict)"("Value"=w329) -> ()  [unwired: 2 in, 2 out]
        n248 = property on="Step size (um)" class="DigNum (strict)"("Value"=w328) -> ()  [unwired: 2 in, 2 out]
        n249 = property on="Z correction factor" class="DigNum (strict)"("Value"=w327) -> ()  [unwired: 2 in, 2 out]
        n250 = property on="ZLUT Start piezo Z" class="DigNum (strict)"("Value"=w325) -> ()  [unwired: 2 in, 2 out]
        n251 = property on="Pixel size (nm)" class="DigNum (strict)"("Value"=w323) -> ()  [unwired: 2 in, 2 out]
        n252 = local write "Use LUT scale for Z"(w293) -> ()
        n253 = String To Path(string=w312) -> (path=w311:path)
        n254 = String To Path(string=w313) -> (path=w310:path)
        n255 = local write "Use gain/offset \ncorrection?"(w314) -> ()
        n256 = property on="Bead index" class="DigNum (strict)"("Maximum"=w316, "Minimum"=0.0 ("Data Entry Limits:Minimum")) -> ()  [unwired: 2 in, 2 out]
        n257 = call "TryLoadGainCorrectionImages.vi"("Pixel Calibration Offset Image"=w310, "Pixel Calibration Gain Image"=w311) -> ("-Offset flat"=w298:sgl[], "1/Gain flat"=w301:sgl[], "-Offset"=w303:sgl[][], "Normalized 1/Gain"=w305:sgl[][])  [unwired: 6 in]
        "Normalized 1/Gain" <- w305
        "Offset" <- w303
        n258 = local write "Pixel calibration offset:"(w310) -> ()
        n259 = call <vilib>:"Std Deviation and Variance.vi"("X"=w298) -> ("mean"=→"Mean":dbl, "standard deviation"=→"St. Dev":dbl)  [unwired: 1 in, 1 out]
        n260 = call <vilib>:"Std Deviation and Variance.vi"("X"=w301) -> ("mean"=→"Mean":dbl, "standard deviation"=→"St Dev.":dbl)  [unwired: 1 in, 1 out]
        n261 = Array Max & Min(array=w298) -> (max value=→"Max":sgl, min value=→"Min":sgl)  [unwired: 2 out]
        n262 = local write "Pixel calibration gain:"(w311) -> ()
        n263 = Array Max & Min(array=w301) -> (max value=→"Max":sgl, min value=→"Min":sgl)  [unwired: 2 out]
        n264 = Array Size(array=w305) -> (size(s)=→"Gain image size":i32[])
        n265 = Array Size(array=w303) -> (size(s)=→"Offset image size":i32[])
      }
      event "LUT Inspect": Value Change {
        n266 = event-data() -> ()  [unwired: 1 in, 5 out]
        n267 = vi-ref "LUTInspectionDlg.vi"() -> (w334:refnum<vi>)
        n268 = invoke class="VI (strict)" method="FP.Open"(reference=w334, "Activate"=TRUE ("Activate?"), "State"=T34."Standard") -> ()  [unwired: 2 in, 5 out]
      }
      event "Auto discard": Value Change {
        n269 = event-data() -> ()  [unwired: 1 in, 5 out]
        n270 = local read "Buffer Image"() -> (w336:T1)
        n271 = call "AutoDiscardBeads.vi"("Minimum bead validity"="Minimum bead validity", "Buffer Image"=w336) -> ()  [unwired: 10 in]
      }
      event User Event {
        n272 = event-data() -> ()  [unwired: 1 in, 2 out]
        n273 = global read "GlobalVariables.vi" "MeasureConfig"() -> (w343:T2)
        n274 = Unbundle By Name(w343) -> ("Tracking Config.ZLUT stepsize (um)"=w340:sgl, "Tracking Config.Start piezo Z (um)"=w341:sgl, "ZLUT"=w342:sgl[][][])
        n275 = local read "Bead index"() -> (w344:i32)
        n276 = property on="Z Lookup Table" class="IntGraph (strict)"("YScale.Multiplier"=w340, "YScale.Offset"=w341) -> ()  [unwired: 2 in, 2 out]
        n277 = Index Array(array=w342, index (dim 0)=w344) -> (element=w339:sgl[][])  [unwired: 2 in]
        "Z Lookup Table" <- w339
        n278 = call "LUTPlane2PlaneDist.vi"("ZLUT"=w339) -> ("min index"=→"LUT minimum\nplane index":i32, "min diff"=→"LUT minimum\nplane difference":sgl)  [unwired: 6 in, 3 out]
      }
      event "Save beadlist", "Load beadlist": Value Change {
        n279 = event-data() -> ()  [unwired: 1 in, 5 out]
        n280 = global read "GlobalVariables.vi" "MeasureConfig"() -> (w346:T2)
        n281 = Unbundle By Name(w346) -> ("Bead locations"=w352:cluster{"X":i32, "Y":i32}[])
        n282 = call "GetExperimentPaths.vi"("MeasureConfig"=w346) -> ("[base]\\beadlist.txt"=w351:path)  [unwired: 6 in, 8 out]
        n283 = call "SaveOrLoadBeadlist.vi"("beadlist filename"=w351, "Load beadlist"="Load beadlist", "Bead locations (input)"=w352) -> ("Bead locations (output)"=w350:cluster{"X":i32, "Y":i32}[])  [unwired: 8 in]
        n284 = Unbundle By Name(w347) -> ("UpdateUI"=w349:refnum<user-event>)
        n285 = Bundle By Name(cluster=w346, "Bead locations"=w350) -> (w345:T2)
        n286 = global write "GlobalVariables.vi" "MeasureConfig"(w345) -> ()
        n287 = Generate User Event(user event=w349, event data cluster=cluster{"ID":dbl} {"ID"=0.0} ("event data")) -> ()  [unwired: 1 in, 2 out]
      }
    }
    n288 = global read "GlobalVariables.vi" "Quit app"() -> (w106:bool)
  }
  n289 = Unbundle By Name(w1) -> ("User Interface Event Notifier"=w3:refnum<notifier>)
  n290 = flat-sequence {
    tunnel: w5 -> [_]
    frame #0 {
      # "Need to wait for the experiment loop to finish before results\ncan be freed"
      n291 = local read "Running\nexperiment"() -> (w354:bool)
      n292 = case shown="True" w354 {
        frame False {
        }
        frame True {
          n293 = while {
            stop <- w355 continue-if-true
            n294 = local read "Running\nexperiment"() -> (w355:bool)
          }
        }
      }
    }
    frame #1 {
      n295 = call "ToggleMainCameraView.vi"("Enable? (T)"=FALSE) -> ()  [unwired: 11 in]
      n296 = call "SetResultManagerInstance.vi"("ResultManager"=T17 {"InstancePtr"=0}) -> ()  [unwired: 11 in]
    }
  }
  n297 = while {
    tunnel: w4 -> [w364]
    tunnel: w3 -> [w363]
    tunnel: w3 -> [w360]
    stop <- w365 stop-if-true
    # "User Interface command loop. This allows different parts of the program to send \nUI commands by using the User Interface message queue"
    n298 = Get Notifier Status(notifier=w363) -> (# waiting=→"Number of listeners":i32)  [unwired: 1 in, 4 out]
    n299 = Wait on Notification(notifier=w360, timeout in ms (-1)=50) -> (notification=w358:T38, timed out?=w359:bool)  [unwired: 2 in, 2 out]
    n300 = case shown="False" w359 {
      tunnel: w364 -> [w368 _]
      tunnel: w358 -> [w367 _]
      frame False {
        n301 = Unbundle By Name(w367) -> ("Type"=w366:T28)
        n302 = case shown="\"MeasureStart\"" w366 {
          tunnel: w368 -> [w370 _ _ _ w376]
          frame "MeasureConfigUpdated" {
            n303 = Unbundle By Name(w370) -> ("UpdateUI"=w369:refnum<user-event>)
            n304 = Generate User Event(user event=w369, event data cluster=cluster{"ID":dbl} {"ID"=0.0} ("event data")) -> ()  [unwired: 1 in, 2 out]
          }
          frame "MeasureEnd" {
            n305 = local write "Running\nexperiment"(FALSE ("Running\nexperiment")) -> ()
          }
          frame "MeasureStart" {
            n306 = local write "Running\nexperiment"(TRUE ("Running\nexperiment")) -> ()
          }
          frame Default {
          }
          frame "ResultTracesUpdated" {
            n307 = Unbundle By Name(w376) -> ("UpdateTraces"=w375:refnum<user-event>)
            n308 = Generate User Event(user event=w375, event data cluster=cluster{"ID":dbl} {"ID"=0.0} ("event data")) -> ()  [unwired: 1 in, 2 out]
          }
        }
      }
      frame True {
      }
    }
    n309 = global read "GlobalVariables.vi" "Quit app"() -> (w365:bool)
  }
